vi "Get Total Target Flow.vi"(0 "Session Handle in":T1, 11 "error in (no error)":errorcluster) -> (4 "Session Handle out":T1, 6 "Total Target Flow":sgl, 15 "error out":errorcluster)   [LabVIEW 2015, in "Environics.lvclass"]
uses:
  Environics.lvclass
  Typedefs/Session Handle.ctl
  Environics.lvclass/Environics.ctl
  C:/TMflex/Test Fixtures/PAS Calibration/Distributed/EnvComm.dll
  EnvComm.dll
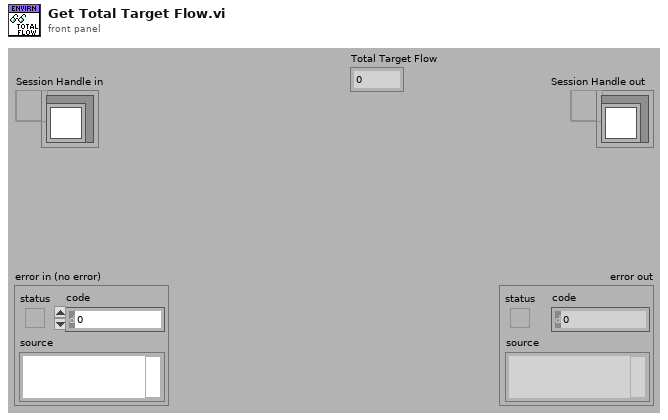
[diagram p1: front panel]
types:
  T1 = typedef "Environics.lvclass/Session Handle.ctl" = refnum<data-value>
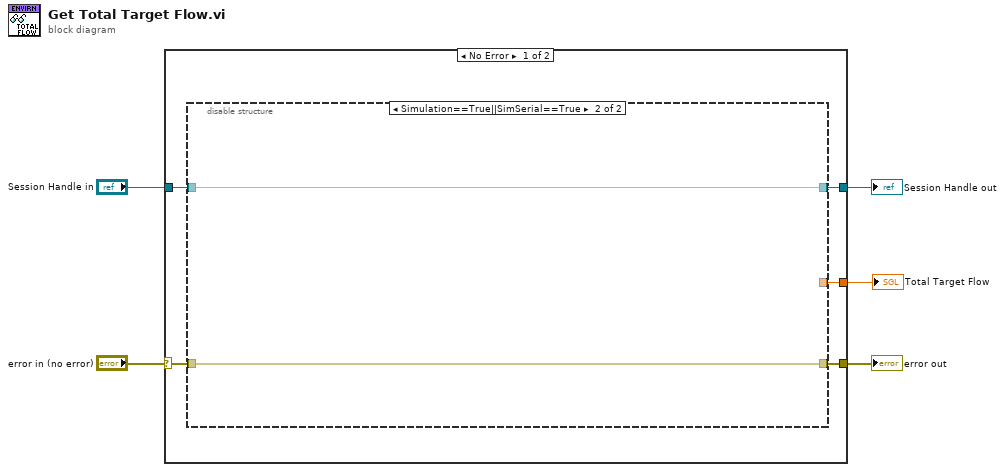
[diagram p0: block diagram]
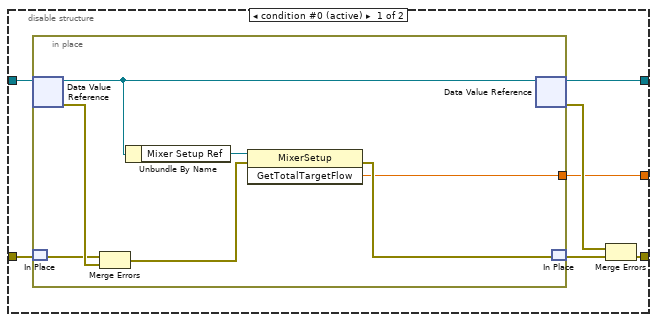
[diagram p2: hidden frame]
diagram:
  n1 = case shown="No Error" "error in (no error)" {
    selector: "error in (no error)" -> [w7 w27]
    tunnel: "Session Handle in" -> [w10 w28]
    tunnel: [w9 w28] -> w4
    tunnel: [w8 w27] -> w3
    tunnel: [w6 _] -> w1
    frame No Error {
      n2 = disable-structure shown="Simulation==True||SimSerial==True" {
        disable-tunnel: w10 -> [w17 w26]
        disable-tunnel: [w16 w26] -> w9
        disable-tunnel: [w15 w25] -> w8
        disable-tunnel: w7 -> [w14 w25]
        disable-tunnel: [w11 _] -> w6
        frame condition #0 (active) {
          n3 = in-place {
            in-place-border: [w18] -> w11
            n4 = in-place-dvr #1(w17) -> (w22:refnum<class "Environics.lvclass">, w24:errorcluster)
            n5 = in-place-match #2(w14) -> (w23:errorcluster)
            n6 = Merge Errors(w23, w24) -> (w20:errorcluster)
            n7 = Unbundle By Name(w22) -> ("Mixer Setup Ref"=w21:refnum<k24>)
            n8 = invoke class="MixerSetup" method="GetTotalTargetFlow"(reference=w21, error in=w20) -> (error out=w19:errorcluster, "GetTotalTargetFlow"=w18:sgl)  [unwired: 1 in, 1 out]
            n9 = in-place-dvr #1(w22) -> (w16:T1, w12:errorcluster)
            n10 = in-place-match #2(w19) -> (w13:errorcluster)
          }
          n11 = Merge Errors(w12, w13) -> (w15:errorcluster)
        }
        frame condition #1 {
        }
      }
    }
    frame Error {
    }
  }
  "Session Handle out" <- w4
  "error out" <- w3
  "Total Target Flow" <- w1
